vi "DataLimit.vi"(3 "Max":dbl, 4 "Data":dbl, 5 "Min":dbl) -> (1 "Data Out":dbl)   [LabVIEW 2018]
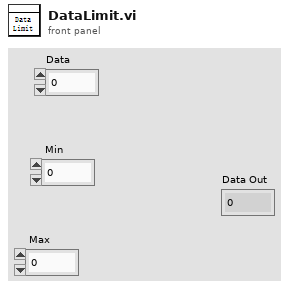
[diagram p1: front panel]
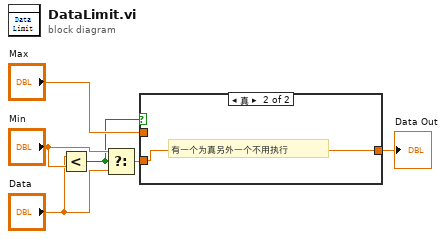
[diagram p0: block diagram]
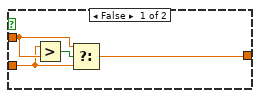
[diagram p2: hidden frame]
diagram:
  n1 = Less?(x="Data", y="Min") -> (x < y?=w1:bool)
  n2 = Select(t="Min", s=w1, f="Data") -> (s? t:f=w3:dbl)
  n3 = case shown="真" w1 {
    tunnel: "Max" -> [w9 _]
    tunnel: w3 -> [w8 w11]
    tunnel: [w7 w11] -> w2
    frame False {
      n4 = Greater?(x=w8, y=w9) -> (0:w10:bool)
      n5 = Select(t=w9, s=w10, f=w8) -> (s? t:f=w7:dbl)
    }
    frame True {
      # "有一个为真另外一个不用执行"
    }
  }
  "Data Out" <- w2
